vi "Maintenance_Modbus.vi"(1 "Maintenance Parameters":T1, 2 "Maintainence position":i32, 3 "Maintenance Hardware Torque":u16, 4 "Maintenance Software Torque":u16, 5 "error in (no error)":errorcluster) -> ()   [LabVIEW 2021]
uses:
  <vilib>/Modbus/master/Modbus Master.lvclass
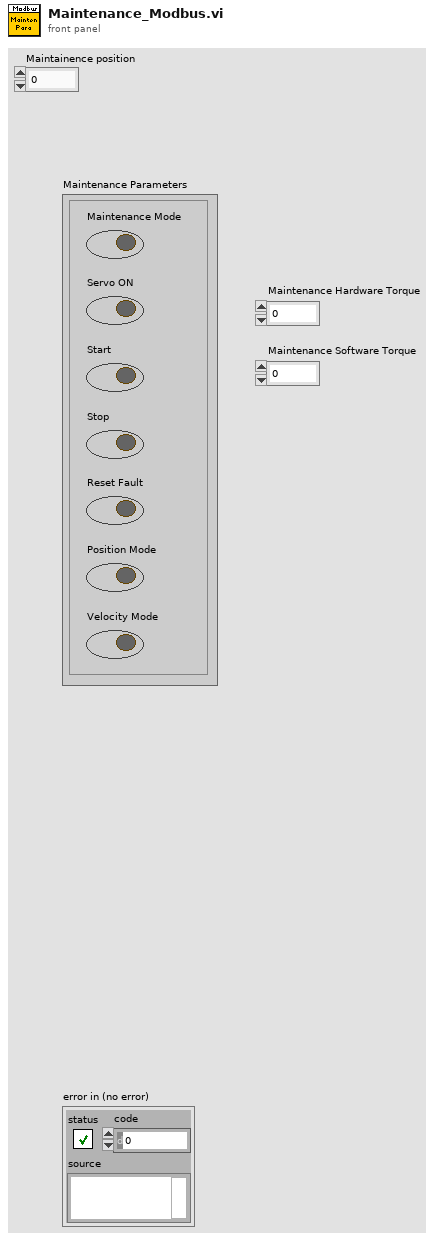
[diagram p1: front panel]
types:
  T1 = cluster{"Maintenance Mode":bool, "Servo ON":bool, "Start":bool, "Stop":bool, "Reset Fault":bool, "Position Mode":bool, "Velocity Mode":bool}
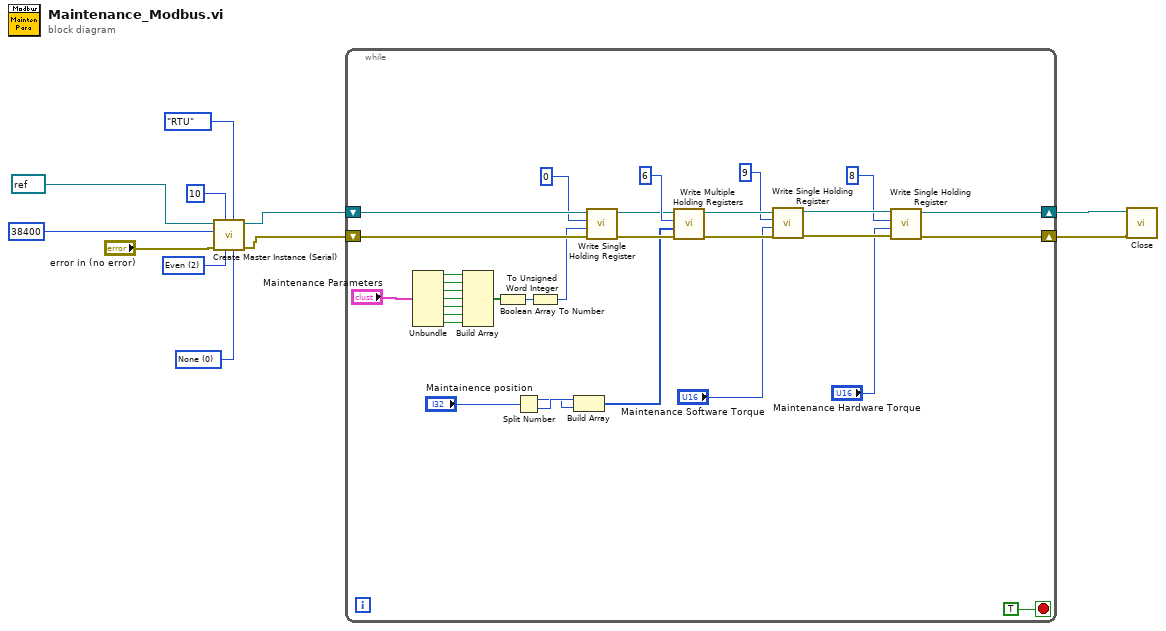
[diagram p0: block diagram]
diagram:
  w3 = u16 0 items=["None", "XON/XOFF", "RTS/CTS", "XON/XOFF & RTS/CTS", "DTR/DSR", "XON/XOFF & DTR/DSR"] ("flow control (None)")
  w4 = u16 2 items=["None", "Odd", "Even"] ("parity (Even)")
  n1 = call <vilib>:"Create Master Instance (Serial).vi"("flow control (None)"=w3, "serial type"=enum16{"RTU", "ASCII"}."RTU", "parity (Even)"=w4, "unit ID"=u8 10, "error in (no error)"="error in (no error)", "baud rate (9600)"=u32 38400, "VISA resource name"=refnum<visa-resource-name> refnum) -> ("error out"=w10:errorcluster, "serial master instance"=w9:refnum<class "Modbus Master.lvclass">)  [unwired: 3 in]
  n2 = while {
    shift-right: [w17] -> w2
    shift-left: w9 -> [w43]
    shift-right: [w18] -> w1
    shift-left: w10 -> [w42]
    stop <- TRUE stop-if-true
    n3 = Unbundle("Maintenance Parameters") -> ("Maintenance Mode"=w39:bool, "Servo ON"=w38:bool, "Start"=w37:bool, "Stop"=w36:bool, "Reset Fault"=w35:bool, "Position Mode"=w34:bool, "Velocity Mode"=w33:bool)
    n4 = Build Array(w39, w38, w37, w36, w35, w34, w33) -> (w32:bool[])
    n5 = Boolean Array To Number(Boolean array=w32) -> (number=w31:u32)
    n6 = Split Number(x="Maintainence position") -> (hi(x)=w12:u16, lo(x)=w13:u16)
    n7 = To Unsigned Word Integer(number=w31) -> (unsigned 16bit integer=w30:u16)
    n8 = Build Array(w13, w12) -> (w14:u16[])
    n9 = call-dynamic "Write Single Holding Register.vi"("error in (no error)"=w42, "holding register value"=w30, "address"=u16 0, "Modbus master in"=w43) -> ("error out"=w27:errorcluster, "Modbus master out"=w28:refnum<class "Modbus Master.lvclass">)  [unwired: 6 in]
    n10 = call-dynamic "Write Multiple Holding Registers.vi"("error in (no error)"=w27, "holding register values"=w14, "starting address"=u16 6, "Modbus master in"=w28) -> ("error out"=w26:errorcluster, "Modbus master out"=w25:refnum<class "Modbus Master.lvclass">)  [unwired: 6 in]
    n11 = call-dynamic "Write Single Holding Register.vi"("error in (no error)"=w26, "holding register value"="Maintenance Software Torque", "address"=u16 9, "Modbus master in"=w25) -> ("error out"=w21:errorcluster, "Modbus master out"=w22:refnum<class "Modbus Master.lvclass">)  [unwired: 6 in]
    n12 = call-dynamic "Write Single Holding Register.vi"("error in (no error)"=w21, "holding register value"="Maintenance Hardware Torque", "address"=u16 8, "Modbus master in"=w22) -> ("error out"=w18:errorcluster, "Modbus master out"=w17:refnum<class "Modbus Master.lvclass">)  [unwired: 6 in]
  }
  n13 = call-dynamic "Close.vi"("error in (no error)"=w1, "Modbus master in"=w2) -> ()  [unwired: 9 in, 1 out]
